vi "Add Status Section.vi"(8 "error in":errorcluster, 11 "custom device in":T1 format="%.0x") -> (0 "error out":errorcluster, 2 "status section":T1 format="%.0x", 3 "custom device out":T1 format="%.0x")   [LabVIEW 2020, in "Ballard MIL-STD-1553 Scripting.lvlib"]
uses:
  Ballard MIL-STD-1553 Scripting.lvlib
  <vilib>/NI VeriStand/Custom Device API/Custom Device Item Ref.ctl
  Constants.vi
  <vilib>/NI VeriStand/Custom Device API/Custom Device API.lvlib
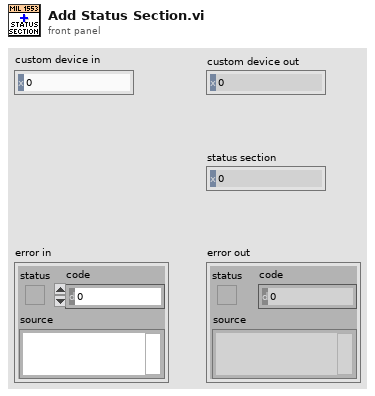
[diagram p1: front panel]
types:
  T1 = typedef "Custom Device API.lvlib/Custom Device Item Ref.ctl" = u64
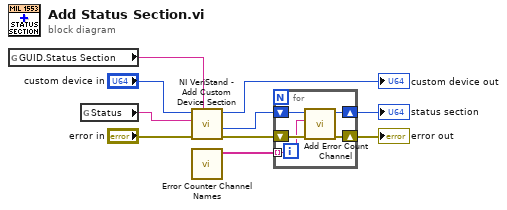
[diagram p0: block diagram]
diagram:
  n1 = global read "Constants.vi" "GUID.Status Section"() -> (w7:string)
  n2 = global read "Constants.vi" "Status"() -> (w6:string)
  n3 = call <vilib>:"NI VeriStand - Add Custom Device Section.vi"("GUID (Default Section)"=w7, "error in (no error)"="error in", "Section Name"=w6, "Parent Ref in"="custom device in") -> ("error out"=w4:errorcluster, "Section Ptr"=w5:T1, "Parent Ref out"=→"custom device out":T1)  [unwired: 4 in, 1 out]
  n4 = call "Error Counter Channel Names.vi"() -> ("error counter channel names"=w1:string[])  [unwired: 11 in]
  n5 = for {
    shift-right: [w13] -> w3
    shift-left: w4 -> [w14]
    shift-right: [w12] -> w2
    shift-left: w5 -> [w15]
    tunnel: w1 -> [w11] mode=indexing
    n6 = call "Add Error Count Channel.vi"("error in"=w14, "error count channel name"=w11, "status section"=w15) -> ("error out"=w13:errorcluster, "error counter channel"=w12:T1)  [unwired: 7 in]
  }
  "error out" <- w3
  "status section" <- w2
